vi "Elevator Controller.vi"(8 "error in (no error)":errorcluster, 11 "View Model":T1) -> (0 "error out":errorcluster)   [LabVIEW 2013]
doc: "Handles all elevator operations."
uses:
  View Model/Controls/View Model.ctl
  Error/Controls/Error Model.ctl
  Error/Controls/Error Types.ctl
  View Model/Controls/Shared Model.ctl
  Controls/Elevator Model.ctl
  Controls/Controller Overhead.ctl
  Controls/Elevator States.ctl
  Controls/Elevator Location.ctl
  Controls/Elevator Command Event.ctl
  Controls/Elevator Commands.ctl
  Configuration/Controls/Configuration Model.ctl
  Configuration/Controls/Configuration Data.ctl
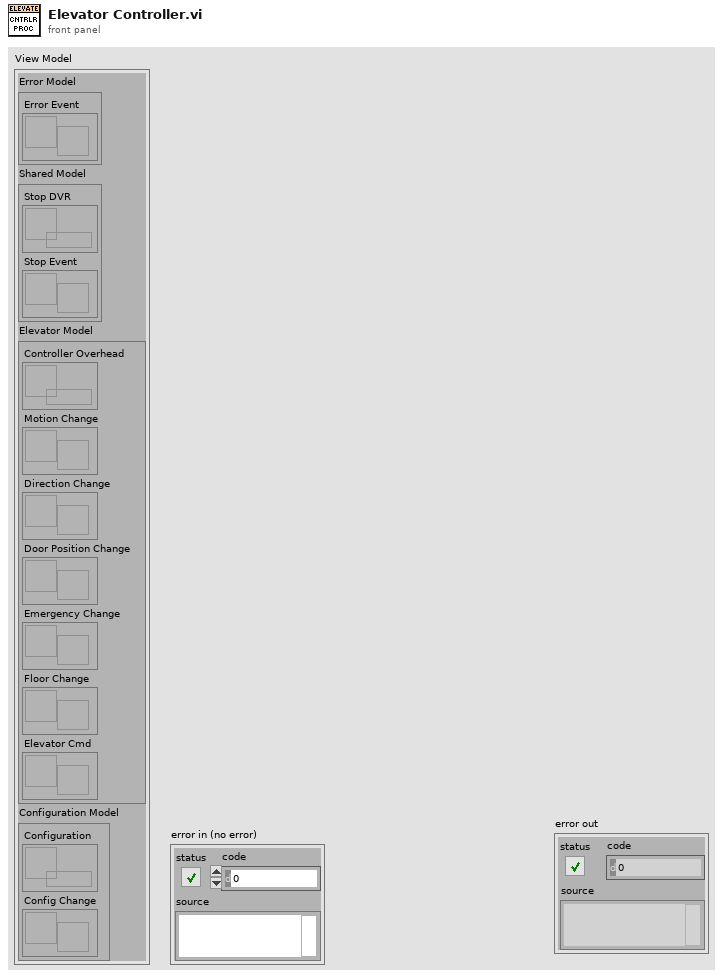
[diagram p1: front panel]
types:
  T1 = typedef "View Model.ctl" = cluster{"Error Model":T2, "Shared Model":T3, "Elevator Model":T4, "Configuration Model":T5}
  T2 = typedef "Error Model.ctl" = cluster{"Error Event":refnum<user-event>}
  T3 = typedef "Shared Model.ctl" = cluster{"Stop DVR":refnum<data-value>, "Stop Event":refnum<user-event>}
  T4 = typedef "Elevator Model.ctl" = cluster{"Controller Overhead":refnum<data-value>, "Motion Change":refnum<user-event>, "Direction Change":refnum<user-event>, "Door Position Change":refnum<user-event>, "Emergency Change":refnum<user-event>, "Floor Change":refnum<user-event>, "Elevator Cmd":refnum<user-event>}
  T5 = typedef "Configuration Model.ctl" = cluster{"Configuration":refnum<data-value>, "Config Change":refnum<user-event>}
  T6 = typedef "Elevator Commands.ctl" = enum16{"Go Up", "Go Down", "Go To Floor", "Emergency", "Open Doors", "Close Doors"}
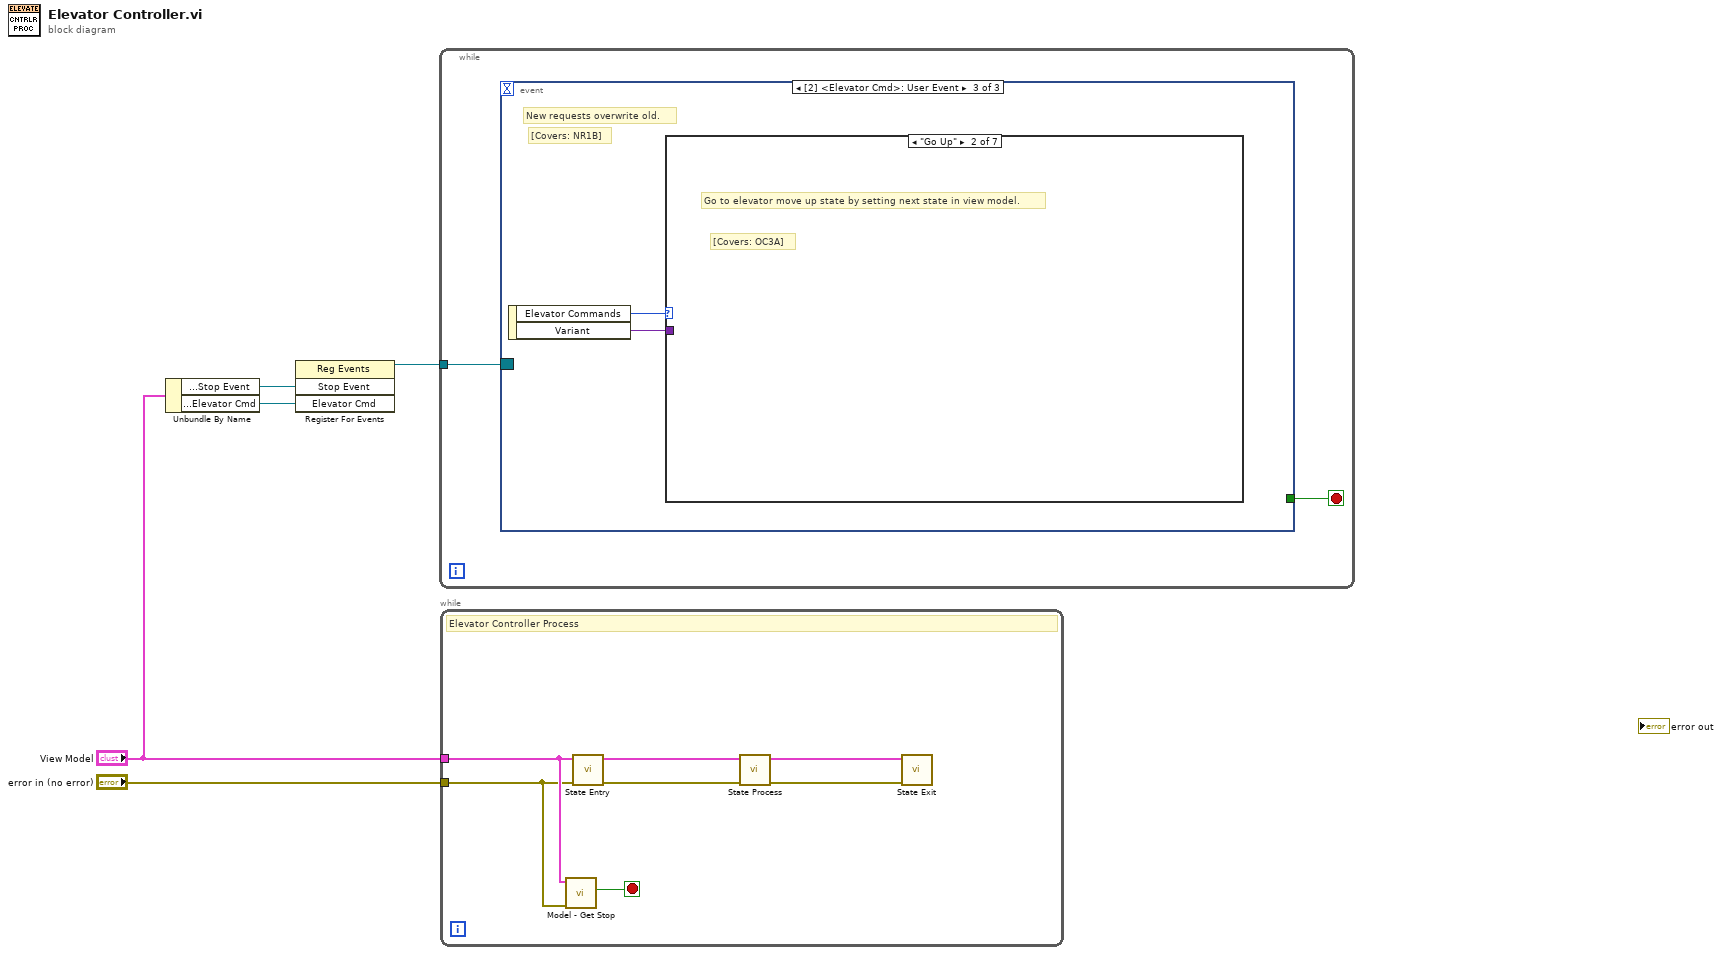
[diagram p0: block diagram]
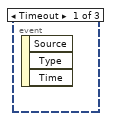
[diagram p2: hidden frame]
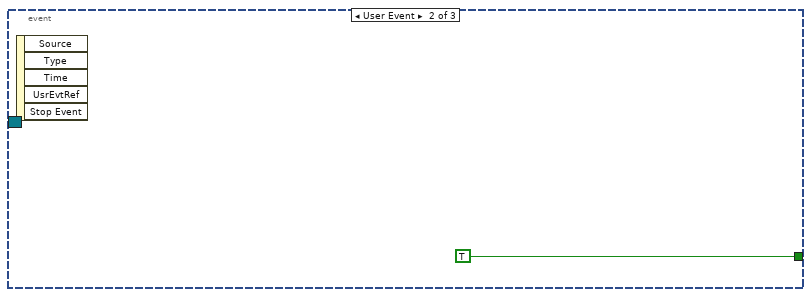
[diagram p3: hidden frame]
diagram:
  n1 = Unbundle By Name("View Model") -> ("Shared Model.Stop Event"=w3:refnum<user-event>, "Elevator Model.Elevator Cmd"=w1:refnum<user-event>)
  n2 = register-events(w3, w1) -> (reference out=w2:refnum<event-registration>)  [unwired: 2 in, 1 out]
  n3 = while {
    tunnel: w2 -> [w7]
    stop <- w6 stop-if-true
    n4 = event shown="[2] <Elevator Cmd>: User Event" {
      selector: w7 -> [_ _ _]
      dyn-events: _ -> [_ _ _]
      timeout: _ -> [_ _ _]
      tunnel: [_ TRUE _] -> w6
      event Timeout {
        n5 = event-data() -> ()  [unwired: 1 in, 3 out]
      }
      event User Event {
        n6 = event-data() -> ()  [unwired: 1 in, 5 out]
      }
      event User Event {
        # "[Covers: NR1B]"
        # "New requests overwrite old."
        n7 = event-data() -> ("Elevator Commands"=w10:T6, "Variant"=w9:variant)  [unwired: 1 in]
        n8 = case shown="\"Go Up\"" w10 {
          tunnel: w9 -> [_ _ _ _ _ _ _]
          frame Default {
          }
          frame "Go Up" {
            # "[Covers: OC3A]"
            # "Go to elevator move up state by setting next state in view model."
          }
          frame "Go Down" {
            # "Go to elevator move down state by setting next state in view model."
          }
          frame "Go To Floor" {
            # "[Covers: WS3]"
            # "[Covers: WS2]"
            # "If on first floor, set open doors to next state, else set travel state."
            # "Go to elevator move up/down state by setting next state in view model."
          }
          frame "Emergency" {
            # "Go to elevator emergency state by setting next state in view model."
          }
          frame "Open Doors" {
            # "Go to elevator open doors state by setting next state in view model."
          }
          frame "Close Doors" {
            # "Go to elevator close doors state by setting next state in view model."
          }
        }
      }
    }
  }
  n9 = while {
    tunnel: "View Model" -> [w13]
    tunnel: "error in (no error)" -> [w12]
    stop <- w11 stop-if-true
    # "Elevator Controller Process"
    n10 = call "Model - Get Stop.vi"("error in (no error)"=w12, "View Model"=w13) -> ("Stop?"=w11:bool)  [unwired: 7 in, 2 out]
    n11 = call "State Entry.vi"("error in (no error)"=w12, "View Model"=w13) -> ("error out"=w16:errorcluster, "View Model"=w17:T1)  [unwired: 8 in]
    n12 = call "State Process.vi"("error in (no error)"=w16, "View Model"=w17) -> ("error out"=w15:errorcluster, "View Model"=w14:T1)  [unwired: 8 in]
    n13 = call "State Exit.vi"("error in (no error)"=w15, "View Model"=w14) -> ()  [unwired: 8 in, 2 out]
  }
